vi "Log If Error.vi"(4 "Event Time":timestamp, 6 "Include Warnings(F)":bool, 7 "Event Level (Error)":T1=enum."Error", 8 "Error In":errorcluster, 9 "Clear After Logging?(F)":bool, 10 "SourceID":string, 11 "Log Instance":refnum<class "LoggerReference.lvclass">) -> (0 "error out":errorcluster, 3 "Log Instance Out":refnum<class "LoggerReference.lvclass">)   [LabVIEW 2017, in "Composed Log.lvlib" / "LoggerReference.lvclass"]
doc: "Log an error event to the logger if an error is present on the error in input. Use the 'Include Warnings' flag to log a warning. \n\nBy default, this method does not clear the incoming error - use the 'Clear After Logging' flag to clear errors."
uses:
  LoggerReference.lvclass
  Types/Log Level.ctl
  LoggerReference.lvclass/LoggerReference.ctl
  Types/Log Packet.ctl
  Remove Stale Logs.vi
  Composed Log.lvlib
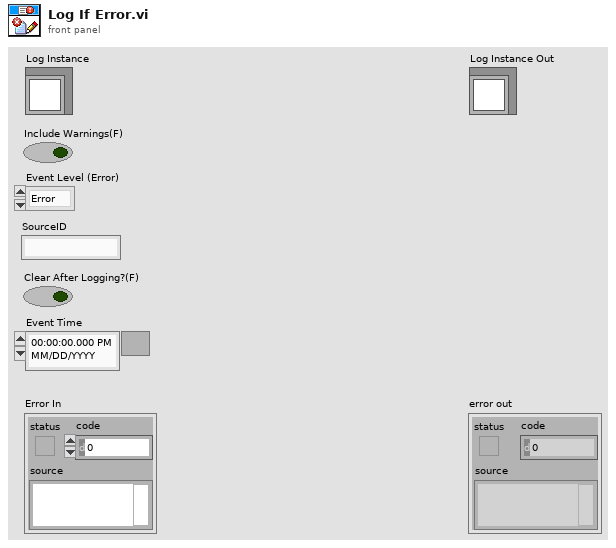
[diagram p1: front panel]
types:
  T1 = typedef "Composed Log.lvlib/Log Level.ctl" = enum16{"Debug", "Info", "Warning", "Error", "Critical"}
  T2 = typedef "Composed Log.lvlib/Log Packet.ctl" = cluster{"Data To Log":string, "Source":string, "Event Level":T1, "Event Time":timestamp}
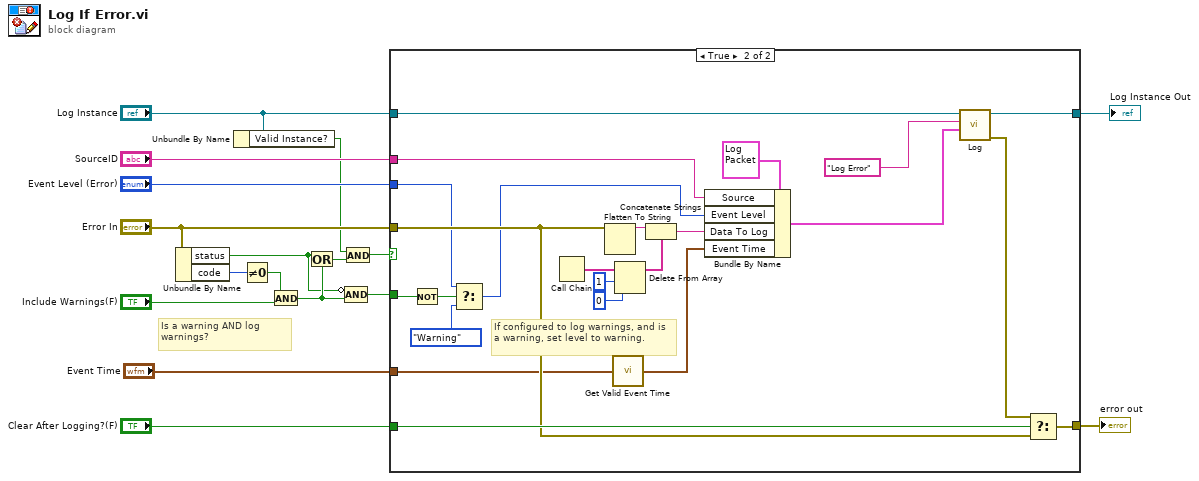
[diagram p0: block diagram]
diagram:
  # "Is a warning AND log warnings?"
  n1 = Unbundle By Name("Error In") -> ("status"=w2:bool, "code"=w13:i32)
  n2 = Unbundle By Name("Log Instance") -> ("Valid Instance?"=w5:bool)
  n3 = Not Equal To 0?(x=w13) -> (x != 0?=w11:bool)
  n4 = And(x=w11, y="Include Warnings(F)") -> (x .and. y?=w3:bool)
  n5 = Or(x=w2, y=w3) -> (x .or. y?=w12:bool)
  n6 = And(x=w5, y=w12) -> (x .and. y?=w6:bool)
  n7 = Compound Arithmetic op=AND(invert w2, w3) -> (w1:bool)
  n8 = case shown="True" w6 {
    tunnel: "SourceID" -> [_ w41]
    tunnel: "Event Level (Error)" -> [_ w25]
    tunnel: [w19 w32] -> w15
    tunnel: "Error In" -> [w19 w33]
    tunnel: "Log Instance" -> [w18 w31]
    tunnel: [w18 w30] -> w9
    tunnel: "Clear After Logging?(F)" -> [_ w34]
    tunnel: "Event Time" -> [_ w21]
    tunnel: w1 -> [_ w26]
    frame False {
      # "No error/not configured to log warnings, do nothing."
    }
    frame True {
      # "If configured to log warnings, and is a warning, set level to warning."
      n9 = Not(x=w26) -> (.not. x?=w22:bool)
      n10 = Select(t=w25, s=w22, f=Log_Level."Warning") -> (s? t:f=w24:T1)
      n11 = Call Chain() -> (call chain=w37:string[])
      n12 = Flatten To String(anything=w33) -> (data string=w40:string)  [unwired: 3 in, 2 out]
      n13 = call "Get Valid Event Time.vi"("Event Time In"=w21) -> ("Event Time Out"=w20:timestamp)
      n14 = Delete From Array(array=w37, length=1, index=0) -> (array with subset deleted=w38:string[])  [unwired: 1 out]
      n15 = Concatenate Strings(w40, w38) -> (w39:string)
      n16 = Bundle By Name(cluster=T2 {"Data To Log"="", "Source"="", "Event Level"=enum."Debug", "Event Time"=timestamp(0 s since 1904-01-01)}, "Source"=w41, "Event Level"=w24, "Data To Log"=w39, "Event Time"=w20) -> (w28:T2)
      n17 = call "Log.vi"("Log Packet"=w28, "Message"="Log Error", "LoggerReference in"=w31) -> ("error out"=w27:errorcluster, "LoggerReference out"=w30:refnum<class "LoggerReference.lvclass">)  [unwired: 7 in]
      n18 = Select(t=w27, s=w34, f=w33) -> (s? t:f=w32:errorcluster)
    }
  }
  "error out" <- w15
  "Log Instance Out" <- w9
